vi "CoerceRange.vi"(8 "error in (no error)":errorcluster, 11 "DAQmx-AI":refnum<class "DAQmx-AI.lvclass">) -> (0 "error out":errorcluster, 2 "Configuration":T1 {"input terminal cfg" items=["Default"=-1, "RSE"=10083, "NRSE"=10078, "Differential"=10106, "Pseudodifferential"=12529]}, 3 "DAQmx-AI out":refnum<class "DAQmx-AI.lvclass">)   [LabVIEW 2016, in "DAQmx-AI.lvclass"]
uses:
  DAQmx-AI.lvclass
  Typedefs/Configuration--Cluster.ctl
  Typedefs/Units -- Enum.ctl
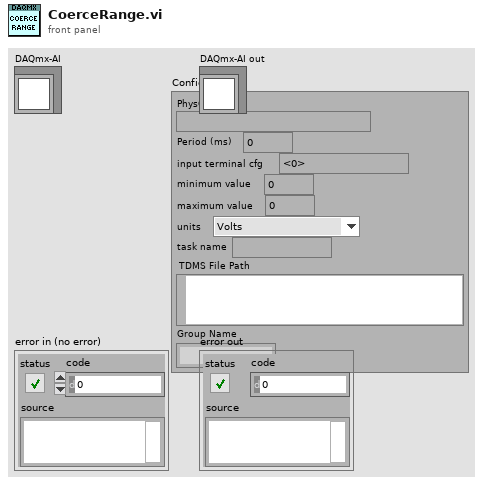
[diagram p1: front panel]
types:
  T1 = typedef "DAQmx-AI.lvclass/Configuration--Cluster.ctl" = cluster{"PhysChan":tag, "Period (ms)":i64, "input terminal cfg":i32, "minimum value":dbl, "maximum value":dbl, "units":T2, "task name":string, "TDMS File Path":path, "Group Name":string}
  T2 = typedef "DAQmx-AI.lvclass/Units -- Enum.ctl" = enum16{"Volts", "Amps", "Deg F", "Deg C", "Deg R", "Kelvins", "Strain", "Ohms", "Hz", "Seconds", "Meters", "Inches", "Degrees", "Radians", "Ticks", "g", "m/s^2", "m/s", "in/s", "Pascals", "Newtons", "Pounds", "kgf", "psi", "bar", "Nm", "oz-in", "lb-in", "lb-ft", "Volts/Volt", "mVolts/Volt", "From TEDS"}
  T3 = typedef "DAQmx-AI.lvclass/Scaling--Cluster.ctl" = cluster{"Scale Name":string, "Scale Type":T4, "Scaled Units":string, "Linear":T5, "Map Range":T6, "Polynomial":T7, "Table":T8}
  T4 = typedef "DAQmx-AI.lvclass/ScalingType--Enum.ctl" = enum16{"No scaling", "Linear", "Map Range", "Polynomial", "Table"}
  T5 = typedef "DAQmx-AI.lvclass/Scaling(Linear)--Cluster.ctl" = cluster{"Slope":dbl, "Intercept":dbl}
  T6 = typedef "DAQmx-AI.lvclass/Scaling(MapRange)--Cluster.ctl" = cluster{"Minimum":dbl, "Maximum":dbl}
  T7 = typedef "DAQmx-AI.lvclass/Scaling(Polynomial)--Cluster.ctl" = cluster{"forward coeff":dbl[], "reverse coeff":dbl[]}
  T8 = typedef "DAQmx-AI.lvclass/Scaling(Table)--Cluster.ctl" = cluster{"scaled values":dbl[], "pres-scaled values":dbl[]}
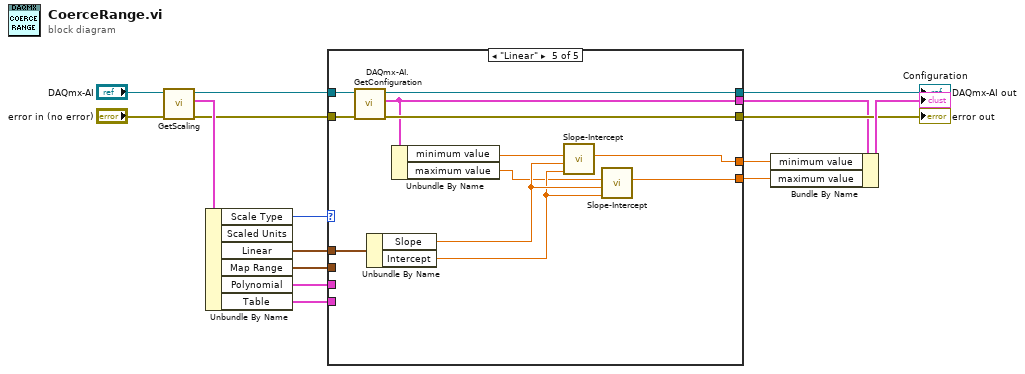
[diagram p0: block diagram]
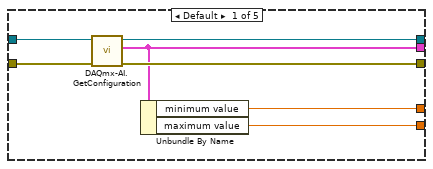
[diagram p2: hidden frame]
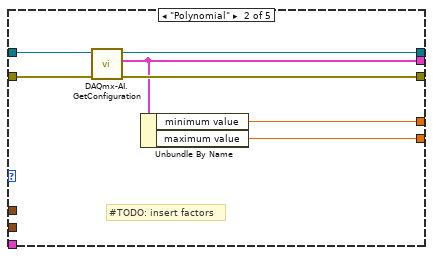
[diagram p3: hidden frame]
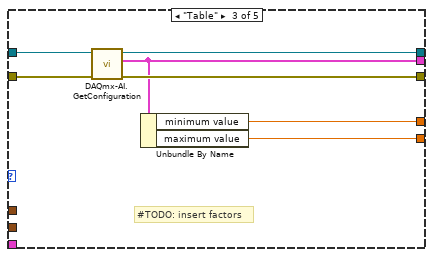
[diagram p4: hidden frame]
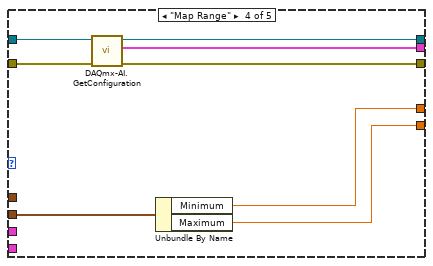
[diagram p5: hidden frame]
diagram:
  n1 = call "GetScaling.vi"("error in (no error)"="error in (no error)", "DAQmx-AI"="DAQmx-AI") -> ("error out"=w14:errorcluster, "Scaling"=w16:T3, "DAQmx-AI out"=w12:refnum<class "DAQmx-AI.lvclass">)  [unwired: 6 in, 1 out]
  n2 = Unbundle By Name(w16) -> ("Scale Type"=w7:T4, "Linear"=w3:T5, "Map Range"=w4:T6, "Polynomial"=w2:T7, "Table"=w1:T8)  [unwired: 1 out]
  n3 = case shown="\"Linear\"" w7 {
    tunnel: w14 -> [w23 w30 w37 w45 w57]
    tunnel: w12 -> [w22 w29 w36 w44 w56]
    tunnel: [w21 w28 w35 w43 w55] -> w10
    tunnel: [w20 w27 w34 w42 w54] -> w9
    tunnel: [w19 w26 w33 w41 w52] -> w8
    tunnel: [w18 w25 w32 w39 w50] -> w6
    tunnel: [w17 w24 w31 w38 w47] -> w5
    tunnel: w4 -> [_ _ _ w40 _]
    tunnel: w3 -> [_ _ _ _ w53]
    tunnel: w2 -> [_ _ _ _ _]
    tunnel: w1 -> [_ _ _ _ _]
    frame Default {
      n4 = call "DAQmx-AI.GetConfiguration.vi"("error in (no error)"=w23, "DAQmx-AI"=w22) -> ("error out"=w21:errorcluster, "Configuration"=w19:T1, "DAQmx-AI out"=w20:refnum<class "DAQmx-AI.lvclass">)  [unwired: 7 in]
      n5 = Unbundle By Name(w19) -> ("minimum value"=w18:dbl, "maximum value"=w17:dbl)
    }
    frame "Polynomial" {
      # "#TODO: insert factors"
      n6 = call "DAQmx-AI.GetConfiguration.vi"("error in (no error)"=w30, "DAQmx-AI"=w29) -> ("error out"=w28:errorcluster, "Configuration"=w26:T1, "DAQmx-AI out"=w27:refnum<class "DAQmx-AI.lvclass">)  [unwired: 7 in]
      n7 = Unbundle By Name(w26) -> ("minimum value"=w25:dbl, "maximum value"=w24:dbl)
    }
    frame "Table" {
      # "#TODO: insert factors"
      n8 = call "DAQmx-AI.GetConfiguration.vi"("error in (no error)"=w37, "DAQmx-AI"=w36) -> ("error out"=w35:errorcluster, "Configuration"=w33:T1, "DAQmx-AI out"=w34:refnum<class "DAQmx-AI.lvclass">)  [unwired: 7 in]
      n9 = Unbundle By Name(w33) -> ("minimum value"=w32:dbl, "maximum value"=w31:dbl)
    }
    frame "Map Range" {
      n10 = call "DAQmx-AI.GetConfiguration.vi"("error in (no error)"=w45, "DAQmx-AI"=w44) -> ("error out"=w43:errorcluster, "Configuration"=w41:T1, "DAQmx-AI out"=w42:refnum<class "DAQmx-AI.lvclass">)  [unwired: 7 in]
      n11 = Unbundle By Name(w40) -> ("Minimum"=w39:dbl, "Maximum"=w38:dbl)
    }
    frame "Linear" {
      n12 = call "DAQmx-AI.GetConfiguration.vi"("error in (no error)"=w57, "DAQmx-AI"=w56) -> ("error out"=w55:errorcluster, "Configuration"=w52:T1, "DAQmx-AI out"=w54:refnum<class "DAQmx-AI.lvclass">)  [unwired: 7 in]
      n13 = Unbundle By Name(w53) -> ("Slope"=w49:dbl, "Intercept"=w48:dbl)
      n14 = Unbundle By Name(w52) -> ("minimum value"=w51:dbl, "maximum value"=w46:dbl)
      n15 = call "Slope-Intercept.vi"("Intercept"=w48, "Slope"=w49, "Value"=w51) -> ("Scaled Value"=w50:dbl)  [unwired: 8 in]
      n16 = call "Slope-Intercept.vi"("Intercept"=w48, "Slope"=w49, "Value"=w46) -> ("Scaled Value"=w47:dbl)  [unwired: 8 in]
    }
  }
  "error out" <- w10
  "DAQmx-AI out" <- w9
  n17 = Bundle By Name(cluster=w8, "minimum value"=w6, "maximum value"=w5) -> (→"Configuration":T1)
